vi "Set Result Collector.vi"(8 "error in (no error)":errorcluster, 10 "Result Collector In":refnum<class "Result Collector.lvclass">, 11 "Execution Profiler In":refnum<class "Execution Profiler.lvclass">) -> (0 "error out":errorcluster, 3 "Execution Profiler Out":refnum<class "Execution Profiler.lvclass">)   [LabVIEW 2020, in "Execution Profiler.lvclass"]
uses:
  Execution Profiler.lvclass
  C:/Users/anton/Documents/GitHub/LUnit/source/Application Framework/Process Classes/Process/Process.lvclass
  Result Collector/Result Collector.lvclass
  Application Framework/Process Classes/Process/Process.lvclass/Process.ctl
  Application Framework/Process Classes/Process/Process.lvclass
  Result Classes/Method Result/Method Result.lvclass
  Result Classes/Test Case Result/Test Case Result.lvclass
  Result Classes/Test Suite Result/Test Suite Result.lvclass
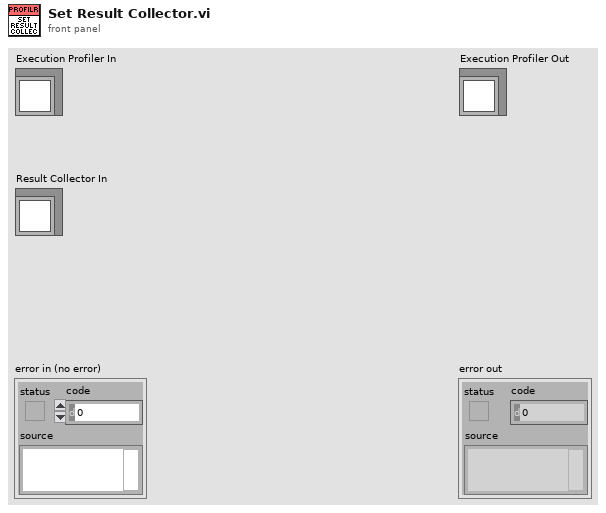
[diagram p1: front panel]
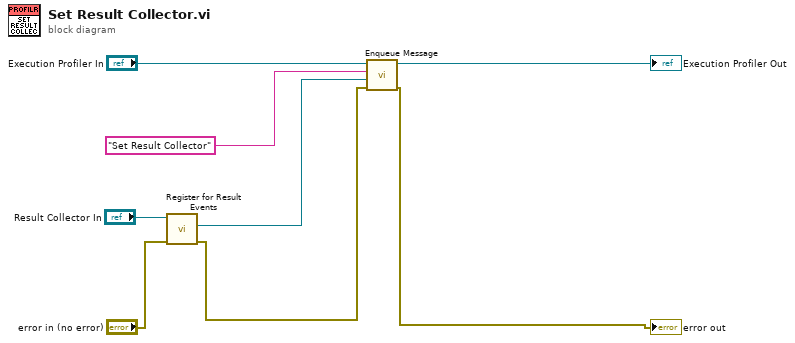
[diagram p0: block diagram]
diagram:
  n1 = call "Register for Result Events.vi"("error in (no error)"="error in (no error)", "Result Collector In"="Result Collector In") -> ("error out"=w3:errorcluster, "Event Registration Refnum"=w7:refnum<event-registration>)  [unwired: 7 in, 1 out]
  n2 = call "Enqueue Message.vi"("error in (no error)"=w3, "Message Data"=w7, "Message"="Set Result Collector", "Process In"="Execution Profiler In") -> ("error out"=→"error out":errorcluster, "Process Out"=→"Execution Profiler Out":refnum<class "Execution Profiler.lvclass">)  [unwired: 6 in]
